vi "1.3.4-Paths.vi"(11 "allowed proximity squared":i16=400) -> ()   [LabVIEW 2010]
uses:
  <vilib>/rvi/DataTransferAndStorage/Container/XNode/niFpgaContainer.xnode
  <vilib>/rvi/FIFO/Fifo_Resource/nirvififoEmulationSetSize.vi
  <vilib>/rvi/DataTransferAndStorage/Container/Common/niFpgaContainerGetUniqueNameForEmu.vi
  1.0-Hindbrain Global.vi
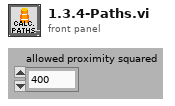
[diagram p1: front panel]
types:
  T1 = enum16{"confirm check sum", "check status byte", "read measured values", "confirm measurement", "confirm command", "read message length", "read address", "wait for \"02\""}
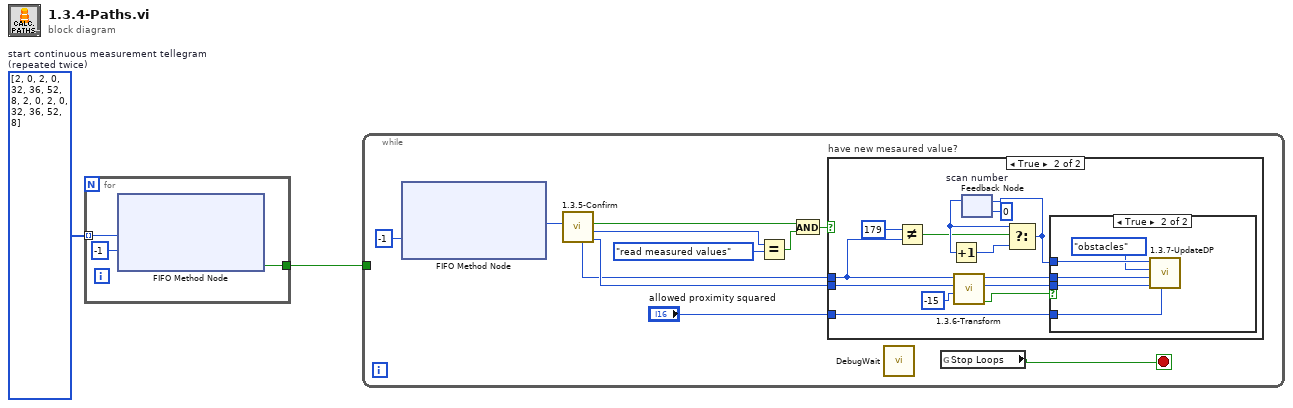
[diagram p0: block diagram]
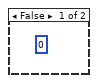
[diagram p2: hidden frame]
diagram:
  w1 = u8[] [2, 0, 2, 0, 32, 36, 52, 8, 2, 0, 2, 0, 32, 36, 52, 8]  # start continuous measurement tellegram (repeated twice)
  n1 = for {
    tunnel: w1 -> [w5] mode=indexing
    tunnel: [w3] -> w2
    n2 = xnode ("FIFO Method Node")("Element"=w5, "Timeout"=-1) -> ("Timed Out?"=w3:bool)  [unwired: 1 in, 1 out]
  }
  n3 = while {
    tunnel: w2 -> [_]
    stop <- w57 stop-if-true
    n4 = xnode ("FIFO Method Node")("Timeout"=-1) -> ("Element"=w67:u8)  [unwired: 1 in, 2 out]
    n5 = call "1.3.5-Confirm.vi"("LIDAR raw data"=w67) -> ("last measured value"=w66:u16, "parser state"=w65:T1, "new value?"=w64:bool, "angle"=w60:u8)  [unwired: 7 in]
    n6 = Equal?(x=w65, y=T1."read measured values" ("parser state")) -> (x = y?=w61:bool)
    n7 = And(x=w64, y=w61) -> (x .and. y?=w63:bool)
    n8 = case "have new mesaured value?" shown="True" w63 {
      tunnel: w66 -> [_ w131]
      tunnel: w60 -> [_ w124]
      tunnel: "allowed proximity squared" -> [_ w119]
      frame False {
        (unwired) u8 0 ("y")
      }
      frame True {
        n9 = Not Equal?(x=u8 179, y=w124) -> (x != y?=w125:bool)
        n10 = call "1.3.6-Transform.vi"("Lidar Vertical Position"=i8 -15, "Lidar Distance"=w131, "Lidar Scan Angle"=w124) -> ("Is object?"=w128:bool, "Robot Y"=w129:i16, "Lidar X = Robot X"=w130:i16)  [unwired: 3 in, 3 out]
        n11 = feedback #1 "scan number"(u8 0 ("y")) -> (w127:u8)
        n12 = Increment(x=w127) -> (x+1=w126:u8)
        n13 = Select(t=w127, s=w125, f=w126) -> (s? t:f=w122:u8)
        n14 = feedback-in #1(w122) -> ()
        n15 = case shown="True" w128 {
          tunnel: w130 -> [_ w136]
          tunnel: w129 -> [_ w135]
          tunnel: w122 -> [_ w134]
          tunnel: w119 -> [_ w132]
          frame False {
          }
          frame True {
            n16 = call "1.3.7-UpdateDP.vi"("allowed proximity squared"=w132, "Robot Y"=w135, "Robot X"=w136, "update lines or objects"=enum16{"lines", "obstacles"}."obstacles", "Scan Number"=w134) -> ()  [unwired: 7 in]
          }
        }
      }
    }
    n17 = call "DebugWait.vi"() -> ()  [unwired: 12 in]
    n18 = global read "1.0-Hindbrain Global.vi" "Stop Loops"() -> (w57:bool)
  }
